vi "SER_RAND.vi"() -> ()   [LabVIEW 2018]
uses:
  Var_serrure.vi
  Var_serrure2.vi
panel:
  out "i":picture
  out "MAX":dbl
  in  "?":bool
  out "Numeric":dbl
  out "CURRENT":dbl
  out "Nombre_entrer":dbl
  in  "?":bool
  out "LED ROUGE":bool
  out "LED VERTE":bool
  in  "Nr3":u8(knob) max=9 step=1 scale=0.0..9.0
  in  "Nr2":u8(knob) max=9 step=1 scale=0.0..9.0
  in  "Nr1":u8(knob) max=9 step=1 scale=0.0..9.0
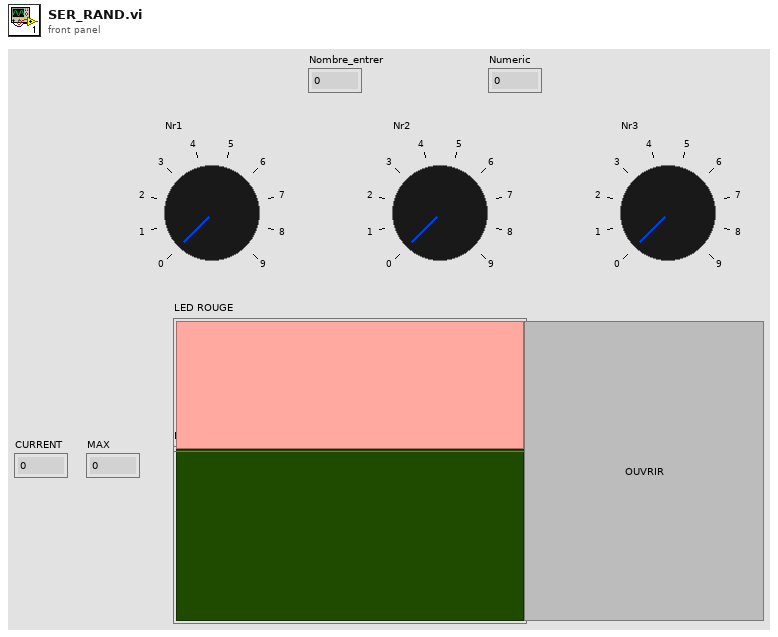
[diagram p1: front panel]
types:
  T1 = typedef "imagedata.ctl" = cluster{"image type":i32, "image depth":i32, "image":u8[], "mask":u8[], "colors":u32[], "Rectangle":cluster{"left":i16, "top":i16, "right":i16, "bottom":i16}}
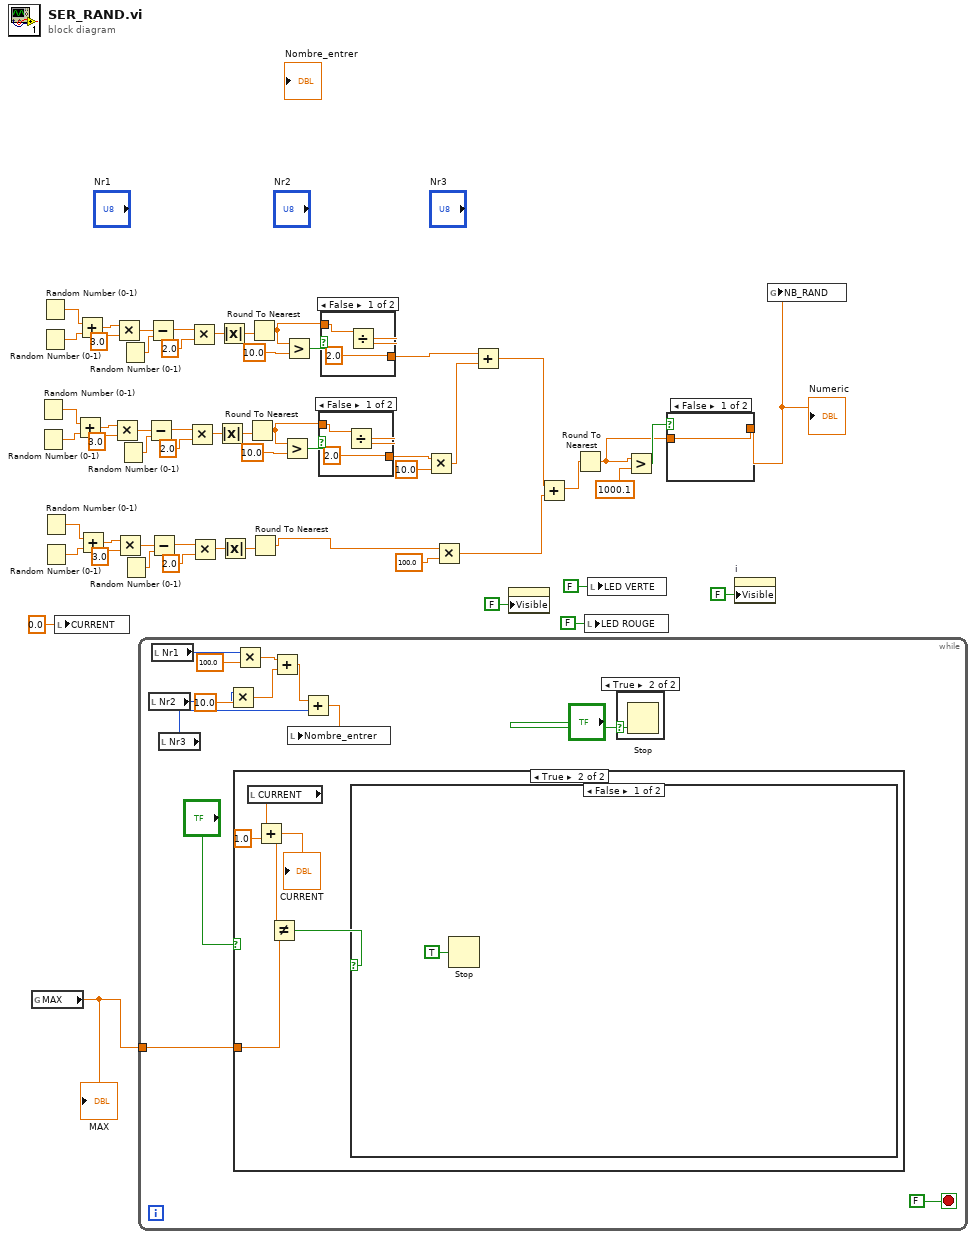
[diagram p0: block diagram]
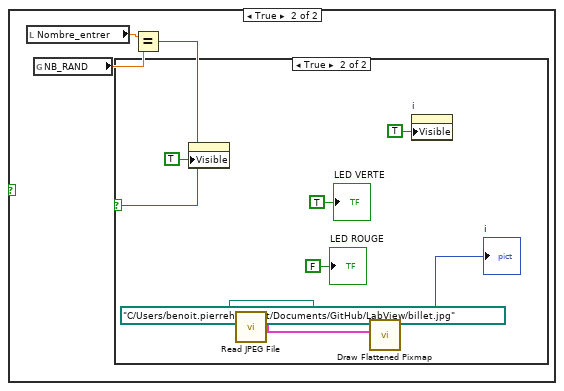
[diagram p4: hidden frame]
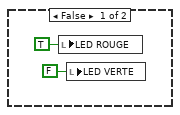
[diagram p5: hidden frame]
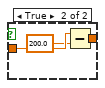
[diagram p6: hidden frame]
diagram:
  n1 = global read "Var_serrure2.vi" "MAX"() -> (w3:dbl)
  "MAX" <- w3
  n2 = Random Number (0-1)() -> (number: 0 to 1=w41:dbl)
  n3 = Random Number (0-1)() -> (number: 0 to 1=w40:dbl)
  n4 = Random Number (0-1)() -> (number: 0 to 1=w55:dbl)
  n5 = Random Number (0-1)() -> (number: 0 to 1=w54:dbl)
  n6 = Random Number (0-1)() -> (number: 0 to 1=w28:dbl)
  n7 = Random Number (0-1)() -> (number: 0 to 1=w27:dbl)
  n8 = local write "CURRENT"(0.0 ("CURRENT")) -> ()
  n9 = Add(x=w41, y=w40) -> (x+y=w39:dbl)
  n10 = Add(x=w55, y=w54) -> (x+y=w53:dbl)
  n11 = Add(x=w28, y=w27) -> (x+y=w26:dbl)
  n12 = Multiply(x=w39, y=3.0) -> (x*y=w37:dbl)
  n13 = Multiply(x=w53, y=3.0) -> (x*y=w51:dbl)
  n14 = Multiply(x=w26, y=3.0) -> (x*y=w24:dbl)
  n15 = Random Number (0-1)() -> (number: 0 to 1=w36:dbl)
  n16 = Random Number (0-1)() -> (number: 0 to 1=w50:dbl)
  n17 = Random Number (0-1)() -> (number: 0 to 1=w23:dbl)
  n18 = while {
    tunnel: w3 -> [w56]
    stop <- FALSE stop-if-true
    n19 = local read "Nr2"() -> (w65:u8)
    n20 = local read "Nr1"() -> (w66:u8)
    n21 = local read "Nr3"() -> (w63:u8)
    n22 = Multiply(x=w65, y=10.0) -> (x*y=w62:dbl)
    n23 = case shown="True" "?" {
      tunnel: w56 -> [_ w74]
      frame False {
      }
      frame True {
        n24 = local read "CURRENT"() -> (w73:dbl)
        n25 = Add(x=w73, y=1.0) -> (x+y=w70:dbl)
        "CURRENT" <- w70
        n26 = Not Equal?(x=w70, y=w74) -> (x != y?=w71:bool)
        n27 = case shown="False" w71 {
          frame False {
            n28 = Stop(stop? (T)=TRUE) -> ()
          }
          frame True {
            n29 = local read "Nombre_entrer"() -> (w77:dbl)
            n30 = global read "Var_serrure.vi" "NB_RAND"() -> (w78:dbl)
            n31 = Equal?(x=w77, y=w78) -> (x = y?=w76:bool)
            n32 = case shown="True" w76 {
              frame False {
                n33 = local write "LED ROUGE"(TRUE ("LED ROUGE")) -> ()
                n34 = local write "LED VERTE"(FALSE ("LED VERTE")) -> ()
              }
              frame True {
                n35 = property class="Bool"("Visible"=TRUE) -> ()  [unwired: 2 in, 2 out]
                n36 = call <vilib>:"Read JPEG File.vi"("path to JPEG file"=path "C:/Users/benoit.pierrehumbert/Documents/GitHub/LabView/billet.jpg") -> ("image data"=w83:T1)  [unwired: 8 in, 2 out]
                n37 = call <vilib>:"Draw Flattened Pixmap.vi"("image data"=w83) -> ("new picture"=→"i":picture)  [unwired: 8 in]
                n38 = property on="i" class="Pict"("Visible"=TRUE) -> ()  [unwired: 2 in, 2 out]
                "LED VERTE" <- TRUE ("LED VERTE")
                "LED ROUGE" <- FALSE ("LED ROUGE")
              }
            }
          }
        }
      }
    }
    n39 = Multiply(x=w66, y=100.0) -> (x*y=w61:dbl)
    n40 = Add(x=w61, y=w62) -> (x+y=w64:dbl)
    n41 = Add(x=w64, y=w63) -> (x+y=w60:dbl)
    n42 = local write "Nombre_entrer"(w60) -> ()
    n43 = case shown="True" "?" {
      selector: "?" -> [_ w69]
      frame False {
      }
      frame True {
        n44 = Stop(stop? (T)=w69) -> ()
      }
    }
  }
  n45 = Subtract(x=w37, y=w36) -> (x-y=w35:dbl)
  n46 = Subtract(x=w51, y=w50) -> (x-y=w49:dbl)
  n47 = Subtract(x=w24, y=w23) -> (x-y=w22:dbl)
  n48 = Multiply(x=w35, y=2.0) -> (x*y=w30:dbl)
  n49 = Multiply(x=w49, y=2.0) -> (x*y=w44:dbl)
  n50 = Multiply(x=w22, y=2.0) -> (x*y=w19:dbl)
  n51 = Absolute Value(x=w30) -> (abs(x)=w32:dbl)
  n52 = Absolute Value(x=w44) -> (abs(x)=w46:dbl)
  n53 = Absolute Value(x=w19) -> (abs(x)=w20:dbl)
  n54 = Round To Nearest(number=w32) -> (nearest integer value=w29:dbl)
  n55 = Round To Nearest(number=w46) -> (nearest integer value=w43:dbl)
  n56 = Round To Nearest(number=w20) -> (nearest integer value=w11:dbl)
  n57 = Greater?(x=w29, y=10.0) -> (0:w31:bool)
  n58 = Greater?(x=w43, y=10.0) -> (0:w45:bool)
  n59 = case shown="False" w31 {
    tunnel: w29 -> [w90 w91]
    tunnel: [w88 w91] -> w17
    frame False {
      n60 = Divide(x=w90, y=2.0) -> (x/y=w88:dbl)
    }
    frame True {
    }
  }
  n61 = case shown="False" w45 {
    tunnel: w43 -> [w94 w95]
    tunnel: [w92 w95] -> w42
    frame False {
      n62 = Divide(x=w94, y=2.0) -> (x/y=w92:dbl)
    }
    frame True {
    }
  }
  n63 = Multiply(x=w17, y=10.0) -> (x*y=w15:dbl)
  n64 = Multiply(x=w11, y=100.0) -> (x*y=w13:dbl)
  n65 = Add(x=w42, y=w15) -> (x+y=w14:dbl)
  n66 = property class="Bool"("Visible"=FALSE) -> ()  [unwired: 2 in, 2 out]
  n67 = Add(x=w14, y=w13) -> (x+y=w12:dbl)
  n68 = Round To Nearest(number=w12) -> (nearest integer value=w8:dbl)
  n69 = local write "LED ROUGE"(FALSE ("LED ROUGE")) -> ()
  n70 = local write "LED VERTE"(FALSE ("LED VERTE")) -> ()
  n71 = Greater?(x=w8, y=1000.1) -> (0:w9:bool)
  n72 = case shown="False" w9 {
    tunnel: w8 -> [w96 w99]
    tunnel: [w96 w97] -> w7
    frame False {
    }
    frame True {
      n73 = Subtract(x=w99, y=200.0) -> (x-y=w97:dbl)
    }
  }
  "Numeric" <- w7
  n74 = property on="i" class="Pict"("Visible"=FALSE) -> ()  [unwired: 2 in, 2 out]
  n75 = global write "Var_serrure.vi" "NB_RAND"(w7) -> ()
